vi "Aircraft RC Override.vi"   [LabVIEW 2014]
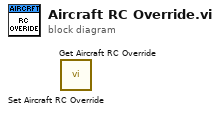
[diagram p0: block diagram]
diagram:
  n1 = call "Set Aircraft RC Override.vi"() -> ()  [unwired: 11 in, 1 out]
  n2 = call "Get Aircraft RC Override.vi"() -> ()  [unwired: 10 in, 2 out]
